vi "sled_test_bench.vi"() -> ()   [LabVIEW 2017]
panel:
  out "rpm_din":dbl
  out "rpm din":dbl(graph)
  in  "tape_space [m]":dbl
  out "distTraveled [m]":dbl
  out "color_dout":dbl
  out "tempIR":dbl(graph)
  out "prox_out_range":bool
  out "prox_min":dbl
  out "prox_max":dbl
  out "prox":dbl
  out "tempIR_max":dbl
  out "tempIR_min":dbl
  out "tempIR":dbl
  out "tempIR_out_range":bool
  out "Edge":bool
  out "rpm_max":dbl
  out "rpm_min":dbl
  # "prox [mm]"
  # "tempIR [c*]"
  # "tempIR_max"
  # "prox_max"
  # "prox_min"
  # "tempIR_min"
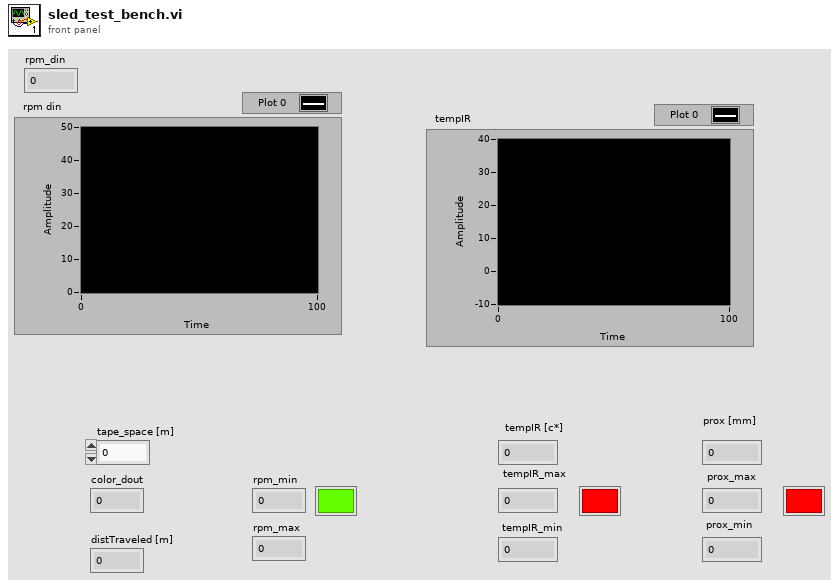
[diagram p1: front panel]
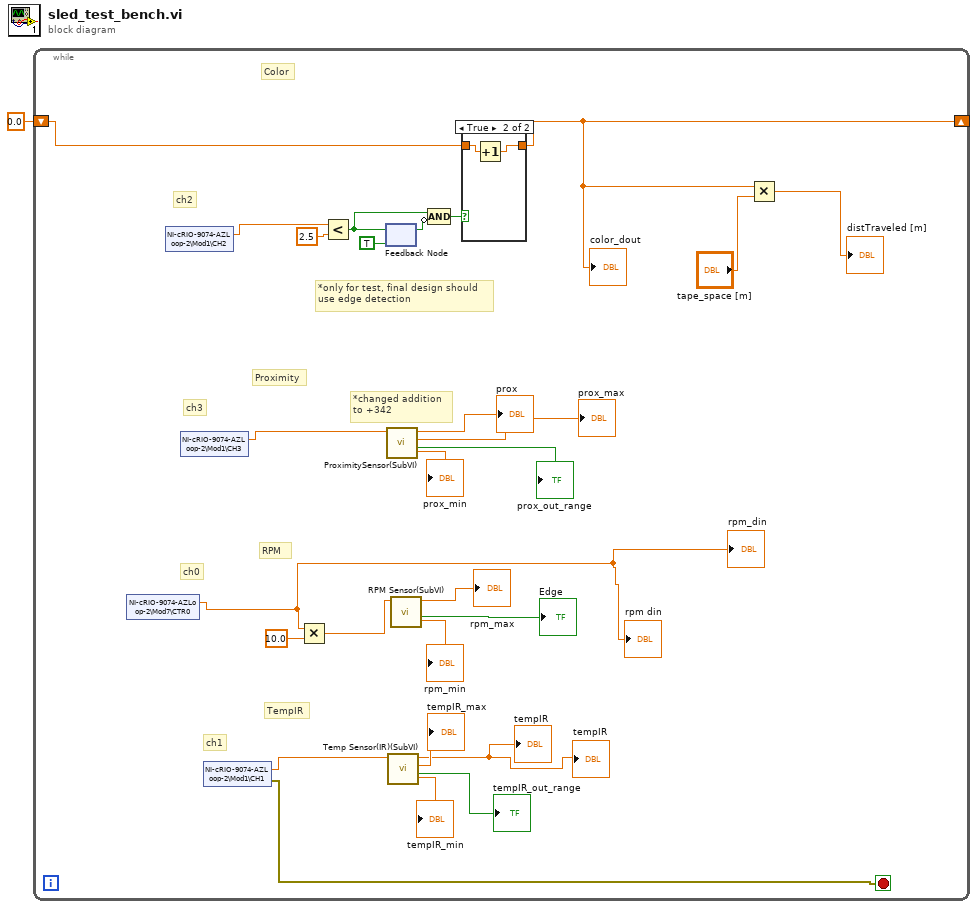
[diagram p0: block diagram]
diagram:
  n1 = while {
    shift-right: [w3] -> _
    shift-left: 0.0 -> [w6]
    stop <- w13 stop-if-true
    # "*changed addition\nto +342"
    # "*only for test, final design should\nuse edge detection"
    # "ch0"
    # "ch1"
    # "ch3"
    # "ch2"
    # "TempIR"
    # "RPM"
    # "Proximity"
    # "Color"
    n2 = shared-variable "NI-cRIO-9074-AZLoop-2\\Mod7\\CTR0"() -> (w2:dbl)  [unwired: 1 in, 1 out]
    "rpm din" <- w2
    "rpm_din" <- w2
    n3 = shared-variable "NI-cRIO-9074-AZLoop-2\\Mod1\\CH2"() -> (w7:dbl)  [unwired: 1 in, 1 out]
    n4 = shared-variable "NI-cRIO-9074-AZLoop-2\\Mod1\\CH3"() -> (w14:dbl)  [unwired: 1 in, 1 out]
    n5 = shared-variable "NI-cRIO-9074-AZLoop-2\\Mod1\\CH1"() -> (w17:dbl, error out=w13:errorcluster)  [unwired: 1 in]
    n6 = Multiply(x=w2, y=10.0) -> (x*y=w15:dbl)
    n7 = Less?(x=w7, y=2.5) -> (x < y?=w9:bool)
    n8 = feedback #1(TRUE) -> (w10:bool)
    n9 = feedback-in #1(w9) -> ()
    n10 = call "ProximitySensor(SubVI).vi"("prox_din"=w14) -> ("prox_out_range"=→"prox_out_range":bool, "prox_max"=→"prox_max":dbl, "prox"=→"prox":dbl, "prox_min"=→"prox_min":dbl)  [unwired: 7 in]
    n11 = call "Temp Sensor(IR)(SubVI).vi"("tempIR_din"=w17) -> ("tempIR_out_range"=→"tempIR_out_range":bool, "tempIR_max"=→"tempIR_max":dbl, "tempIR"=→"tempIR" →"tempIR":dbl, "tempIR_min"=→"tempIR_min":dbl)  [unwired: 7 in]
    n12 = call "RPM Sensor(SubVI).vi"("rpm_din"=w15) -> ("Edge"=→"Edge":bool, "rpm_max"=→"rpm_max":dbl, "rpm_min"=→"rpm_min":dbl)  [unwired: 8 in]
    n13 = Compound Arithmetic op=AND(w9, invert w10) -> (w8:bool)
    n14 = case shown="True" w8 {
      tunnel: w6 -> [w29 w30]
      tunnel: [w29 w31] -> w3
      frame False {
      }
      frame True {
        n15 = Increment(x=w30) -> (x+1=w31:dbl)
      }
    }
    "color_dout" <- w3
    n16 = Multiply(x=w3, y="tape_space [m]") -> (x*y=→"distTraveled [m]":dbl)
  }
